vi "Close Web Service.vi"(8 "error in (no error)":errorcluster, 11 "CheckUserAndEquipmentStatusService refnum":refnum<k24>) -> (0 "error out":errorcluster)   [LabVIEW 2023, in "CheckUserAndEquipmentStatusService.lvlib"]
uses:
  <userlib>/WebService/_CheckUserAndEquipmentStatusService/CheckUserAndEquipmentStatusService.lvlib
  <userlib>/WebService/_CheckUserAndEquipmentStatusService/CheckUserAndEquipmentStatusService.dll
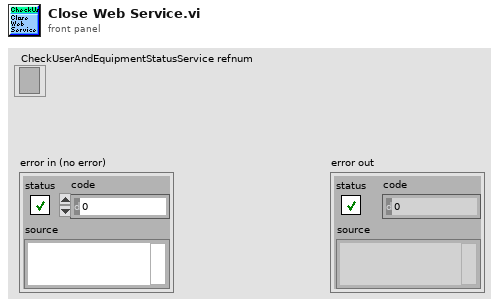
[diagram p1: front panel]
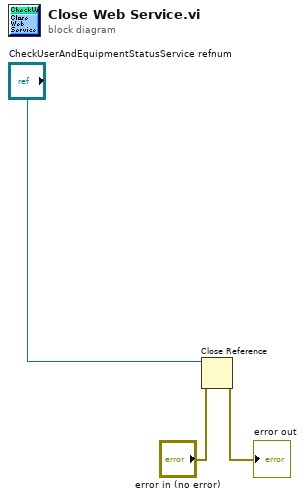
[diagram p0: block diagram]
diagram:
  n1 = Close Reference(reference="CheckUserAndEquipmentStatusService refnum", error in (no error)="error in (no error)") -> (error out=→"error out":errorcluster)
